vi "欧姆龙PLC初始化FansUDP.vi"(9 "端口Port":u16=9600, 11 "PC网络地址 in":u32) -> (0 "网络地址":u32, 2 "PLC初始化结果":bool, 3 "连接ID":refnum<k16>)   [LabVIEW 2014]
panel:
  in  "error in":errorcluster caption="错误输入（无错误）"
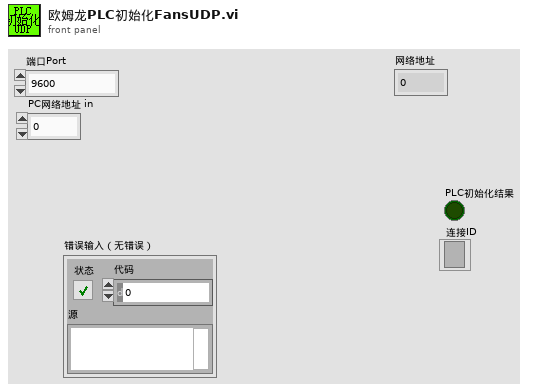
[diagram p1: front panel]
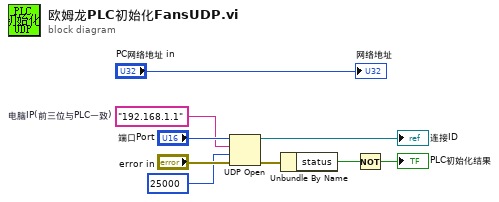
[diagram p0: block diagram]
diagram:
  w1 = "192.168.1.1"  # 电脑IP(前三位与PLC一致)
  n1 = UDP Open(8:"error in", 9:25000 ("超时毫秒(25000)"), 10:w1, 11:"端口Port") -> (port=→"连接ID":refnum<k16>, 0:w7:errorcluster)  [unwired: 1 in, 1 out]
  n2 = Unbundle By Name(w7) -> ("status"=w6:bool)
  n3 = Not(x=w6) -> (.not. x?=→"PLC初始化结果":bool)
  "网络地址" <- "PC网络地址 in"
